vi "Read Default Values from Disk.vi"(0 "reference in":refnum<class "Generic Utilities.lvclass">, 5 "error in (no error)":errorcluster, 6 "AppData Option":T1(ring), 7 "Control Label":string, 9 "Caption":string) -> (13 "Value (XML String)":string, 14 "reference out":refnum<class "Generic Utilities.lvclass">, 19 "error out":errorcluster)   [LabVIEW 2020, in "Generic Utilities.lvclass"]
uses:
  Generic Utilities.lvclass
  <vilib>/Utility/sysdir.llb/System Directory Type.ctl
  <vilib>/Utility/xml.llb/Read From XML File(string).vi
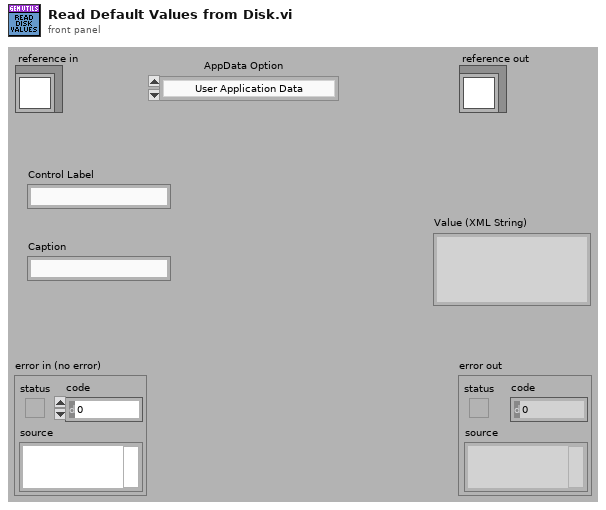
[diagram p1: front panel]
types:
  T1 = enum16{"User Application Data", "Public Application Data"}
  T2 = typedef "Generic Utilities.lvclass/ObjectAttributes.ctl" = cluster{"GUI Parameters":T3, "State Machine Control":cluster{"Timeout":i32, "State Queue":string[], "State History":string[], "State History Length":i32}, "Logging File Path":path, "OBJ not a refnum?":bool, "Timer Start":timestamp, "FP Refnums":T4}
  T3 = typedef "Generic Utilities.lvclass/GUI Parameters.ctl" = cluster{"Application Name":string, "GUI VI Ref":refnum<vi>, "Close Panel?":bool, "Message Window ref":refnum<vi>, "Version #":string}
  T4 = typedef "Generic Utilities.lvclass/FP Refnums.ctl" = cluster{"Panel refnum":refnum<vi>, "Control Labels":string[], "Refnums":refnum<vi>[]}
  T5 = typedef "System Directory Type.ctl" = i32
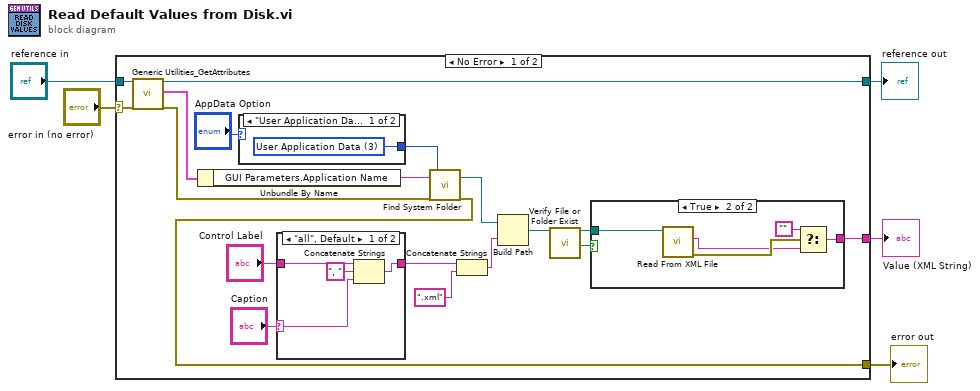
[diagram p0: block diagram]
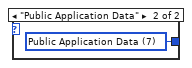
[diagram p2: hidden frame]
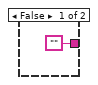
[diagram p4: hidden frame]
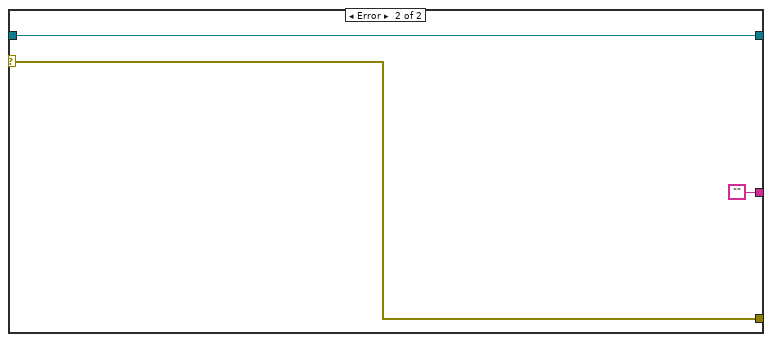
[diagram p5: hidden frame]
diagram:
  n1 = case shown="No Error" "error in (no error)" {
    selector: "error in (no error)" -> [w24 w40]
    tunnel: [w8 w40] -> w4
    tunnel: [w23 w39] -> w2
    tunnel: "reference in" -> [w21 w39]
    tunnel: [w10 ""] -> w1
    frame No Error {
      n2 = call "Generic Utilities_GetAttributes.vi"("reference in"=w21, "error in (no error)"=w24) -> ("reference out"=w23:refnum<class "Generic Utilities.lvclass">, "attributes"=w22:T2, "error out"=w14:errorcluster)  [unwired: 14 in, 1 out]
      n3 = Unbundle By Name(w22) -> ("GUI Parameters.Application Name"=w15:string)
      n4 = case shown="\"User Application Data\", Default" "AppData Option" {
        tunnel: [w25 w26] -> w6
        frame "User Application Data", Default {
          w25 = T5 3 items=["User Home"=0, "User Desktop"=1, "User Documents"=2, "User Application Data"=3, "User Preferences"=4, "User Temporary"=5, "Public Documents"=6, "Public Application Data"=7, "Public Preferences"=8, "Public Cache"=13, "System Core Libraries"=9, "System Installed Libraries"=10, "Application Files"=11, "Boot Volume Root"=12] ("system directory type")
        }
        frame "Public Application Data" {
          w26 = T5 7 items=["User Home"=0, "User Desktop"=1, "User Documents"=2, "User Application Data"=3, "User Preferences"=4, "User Temporary"=5, "Public Documents"=6, "Public Application Data"=7, "Public Preferences"=8, "Public Cache"=13, "System Core Libraries"=9, "System Installed Libraries"=10, "Application Files"=11, "Boot Volume Root"=12] ("system directory type")
        }
      }
      n5 = case shown="\"all\", Default" "Caption" {
        selector: "Caption" -> [w27 _]
        tunnel: [w30 w31] -> w17
        tunnel: "Control Label" -> [w29 w31]
        frame "all", Default {
          n6 = Concatenate Strings(w29, ", " ("string"), w27) -> (w30:string)
        }
        frame "" {
        }
      }
      n7 = call "Find System Folder.vi"("Application Name"=w15, "error in (no error)"=w14, "system directory type"=w6) -> ("System Folder"=w9:path, "error out"=w8:errorcluster)  [unwired: 15 in]
      n8 = Concatenate Strings(w17, ".xml" ("string")) -> (w19:string)
      n9 = Build Path(base path=w9, name or relative path=w19) -> (appended path=w12:path)
      n10 = call "Verify File or Folder Exist.vi"("path"=w12) -> ("dup path"=w13:path, "file or folder exists?"=w11:bool)  [unwired: 16 in, 1 out]
      n11 = case shown="True" w11 {
        tunnel: w13 -> [_ w37]
        tunnel: ["" w34] -> w10
        frame False {
        }
        frame True {
          n12 = call-poly <vilib>:"Read From XML File.vi"("XML File Path"=w37) -> ("error out"=w36:errorcluster, "XML Elements"=w35:string)  [unwired: 8 in, 1 out]
          n13 = Select(t="", s=w36, f=w35) -> (s? t:f=w34:string)
        }
      }
    }
    frame Error {
    }
  }
  "error out" <- w4
  "reference out" <- w2
  "Value (XML String)" <- w1
